vi "publish.vi"(0 "HGF_PVPublisher":refnum<class "HGF_PVPublisher.lvclass">, 1 "typeDescriptor":string, 2 "data":variant, 3 "timeout in ms (-1)":i32, 5 "error in (no error)":errorcluster) -> (14 "dup HGF_PVPublisher":refnum<class "HGF_PVPublisher.lvclass">, 16 "rawData":variant, 17 "timed out?":bool, 19 "error out":errorcluster)   [LabVIEW 2014, in "HGF_BaseClasses.lvlib" / "HGF_PVPublisher.lvclass"]
uses:
  HGF_PVPublisher.lvclass
  HGF_PVBase/HGF_PVBase.lvclass
  HGF_PVDataConverter/HGF_PVDataConverter.lvclass
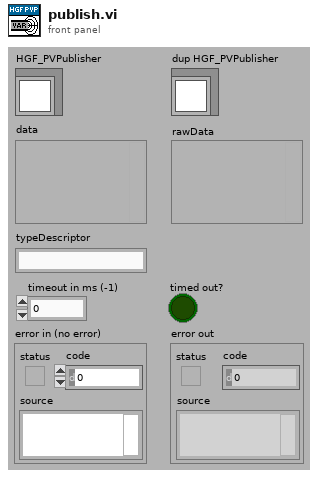
[diagram p1: front panel]
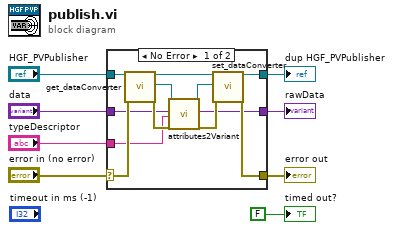
[diagram p0: block diagram]
diagram:
  n1 = case shown="No Error" "error in (no error)" {
    selector: "error in (no error)" -> [w14 w23]
    tunnel: [w13 w23] -> w7
    tunnel: [w20 w22] -> w5
    tunnel: "HGF_PVPublisher" -> [w19 w22]
    tunnel: "data" -> [w12 w21]
    tunnel: "typeDescriptor" -> [w11 _]
    tunnel: [w9 w21] -> w2
    frame No Error {
      n2 = call "get_dataConverter.vi"("HGV_PVBase"=w19, "error in (no error)"=w14) -> ("dup HGV_PVBase"=w18:refnum<class "HGF_PVPublisher.lvclass">, "HGF_PVDataConverter"=w17:refnum<class "HGF_PVDataConverter.lvclass">, "error out"=w16:errorcluster)  [unwired: 15 out]
      n3 = call-dynamic "attributes2Variant.vi"("HGF_PVDataConverter"=w17, "Parameter"=w12, "typeDescriptor"=w11, "error in (no error)"=w16) -> ("HGF_PVDataConverter"=w10:refnum<class "HGF_PVDataConverter.lvclass">, "rawData"=w9:variant, "error out"=w15:errorcluster)  [unwired: 13 out]
      n4 = call "set_dataConverter.vi"("HGV_PVBase"=w18, "HGF_PVDataConverter"=w10, "error in (no error)"=w15) -> ("dup HGV_PVBase"=w20:refnum<class "HGF_PVPublisher.lvclass">, "error out"=w13:errorcluster)  [unwired: 15 out]
    }
    frame Error {
    }
  }
  "error out" <- w7
  "dup HGF_PVPublisher" <- w5
  "rawData" <- w2
  "timed out?" <- FALSE ("timed out?")
